vi "Define Default Paths.vi"() -> ()   [LabVIEW 2026]
uses:
  Measurement Paths Cluster.ctl
  Hardware Paths Cluster.ctl
  <vilib>/Utility/config.llb/Write Key (Boolean).vi
  <userlib>/_OpenG.lib/file/file.llb/Compare Two Paths - Scalar__ogtk.vi
  <vilib>/Utility/config.llb/NI_LVConfig.lvlib
  Controller/Server Controller.lvclass
panel:
  in  "Measurement Folder":path=path "C:/Users/ekerry/Projects/Measurement Utility/Source/Framework/Measurements"
  in  "Hardware Folder":path=path "C:/Users/ekerry/Projects/Measurement Utility/Source/Framework/Installed Hardware"
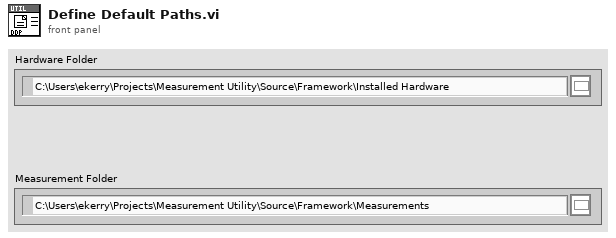
[diagram p1: front panel]
types:
  T1 = typedef "Hardware Paths Cluster.ctl" = cluster{"Paths":path[]}
  T2 = typedef "Measurement Paths Cluster.ctl" = cluster{"Paths":path[]}
  T3 = typedef "NI_LVConfig.lvlib/Config Data RefNum.ctl" = refnum<k1>
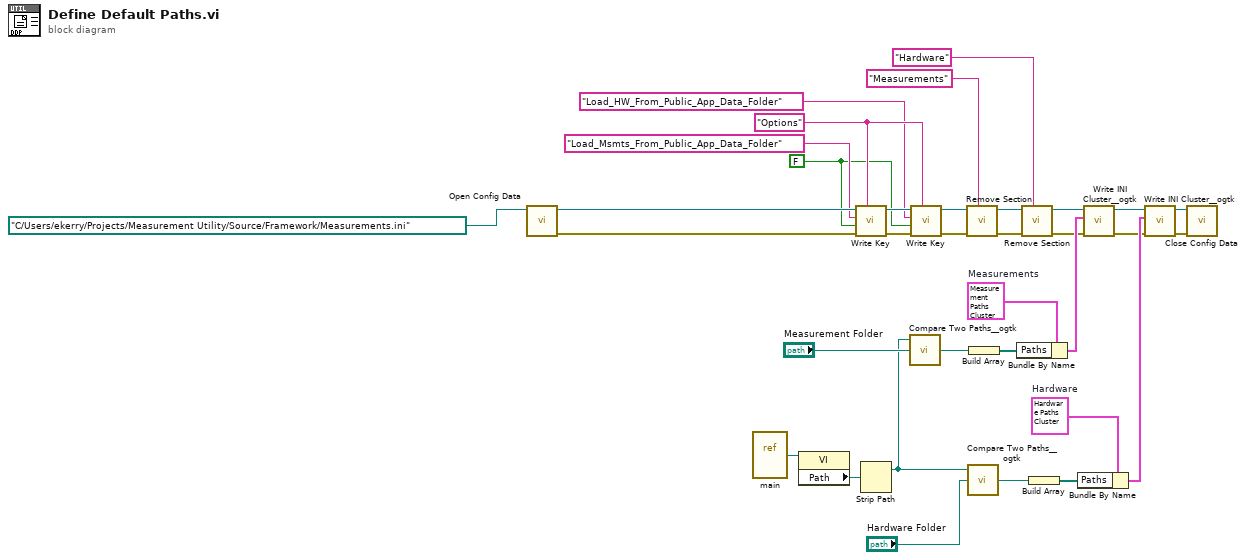
[diagram p0: block diagram]
diagram:
  w2 = FALSE ("value")
  w3 = "Options" ("section")
  w28 = T1 {"Paths"=[path "C:/Users/ekerry/Projects/Measurement Utility/Source/Framework/Installed Hardware"]}  # Hardware
  w30 = T2 {"Paths"=[path "C:/Users/ekerry/Projects/Measurement Utility/Source/Framework/Measurements"]}  # Measurements
  n1 = call <vilib>:"Open Config Data.vi"("configuration file path"=path "C:/Users/ekerry/Projects/Measurement Utility/Source/Framework/Measurements.ini") -> ("error out"=w5:errorcluster, "refnum"=w12:T3)  [unwired: 8 in, 1 out]
  n2 = vi-ref "main.vi"() -> (w31:refnum<vi>)
  n3 = property class="VI"(reference=w31) -> ("Path"=w20:path)  [unwired: 1 in, 2 out]
  n4 = call-poly <vilib>:"Write Key.vi"("section"=w3, "error in (no error)"=w5, "value"=w2, "key"="Load_Msmts_From_Public_App_Data_Folder", "refnum"=w12) -> ("error out"=w14:errorcluster, "refnum out"=w13:T3)  [unwired: 4 in, 1 out]
  n5 = Strip Path(path=w20) -> (stripped path=w19:path)  [unwired: 1 out]
  n6 = call-poly <userlib>:"Compare Two Paths__ogtk.vi"("path2"="Measurement Folder", "path1"=w19) -> ("relative path from 1 to 2"=w25:path)  [unwired: 1 in, 2 out]
  n7 = call-poly <vilib>:"Write Key.vi"("section"=w3, "error in (no error)"=w14, "value"=w2, "key"="Load_HW_From_Public_App_Data_Folder", "refnum"=w13) -> ("error out"=w10:errorcluster, "refnum out"=w11:T3)  [unwired: 4 in, 1 out]
  n8 = call <vilib>:"Remove Section.vi"("section"="Measurements" ("float number format (optional)"), "error in (no error)"=w10, "refnum"=w11) -> ("error out"=w9:errorcluster, "refnum out"=w18:T3)  [unwired: 6 in, 1 out]
  n9 = call-poly <userlib>:"Compare Two Paths__ogtk.vi"("path2"="Hardware Folder", "path1"=w19) -> ("relative path from 1 to 2"=w23:path)  [unwired: 1 in, 2 out]
  n10 = Build Array(w25) -> (w24:path[])
  n11 = Bundle By Name(cluster=w30, "Paths"=w24) -> (w29:T2)
  n12 = call <vilib>:"Remove Section.vi"("section"="Hardware" ("float number format (optional)"), "error in (no error)"=w9, "refnum"=w18) -> ("error out"=w8:errorcluster, "refnum out"=w17:T3)  [unwired: 6 in, 1 out]
  n13 = Build Array(w23) -> (w22:path[])
  n14 = Bundle By Name(cluster=w28, "Paths"=w22) -> (w27:T1)
  n15 = call <userlib>:"Write INI Cluster__ogtk.vi"("error in (no error)"=w8, "INI Fomatted Cluster"=w29, "refnum"=w17) -> ("error out"=w7:errorcluster, "dup refnum"=w33:T3)  [unwired: 7 in]
  n16 = call <userlib>:"Write INI Cluster__ogtk.vi"("error in (no error)"=w7, "INI Fomatted Cluster"=w27, "refnum"=w33) -> ("error out"=w6:errorcluster, "dup refnum"=w32:T3)  [unwired: 7 in]
  n17 = call <vilib>:"Close Config Data.vi"("error in (no error)"=w6, "refnum"=w32) -> ()  [unwired: 8 in, 2 out]
